vi "Create Response.vi"(8 "error in (no error)":errorcluster, 11 "message refnum in":T1 format="%.0x") -> (0 "error out":errorcluster, 2 "response refnum":T1=18446744073709551615 format="%.0x", 3 "message refnum out":T1 format="%.0x")   [LabVIEW 2020, in "Instrument Addon Scripting API.lvlib"]
doc: "Creates a Response section to the specified message. An error will occur if the refnum does not match an existing message."
uses:
  Instrument Addon Scripting API.lvlib
  <vilib>/NI VeriStand/Custom Device API/Custom Device Item Ref.ctl
  <vilib>/NI VeriStand/Custom Device API/Custom Device API.lvlib
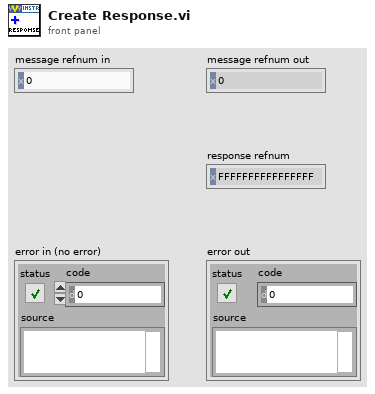
[diagram p1: front panel]
types:
  T1 = typedef "Custom Device API.lvlib/Custom Device Item Ref.ctl" = u64
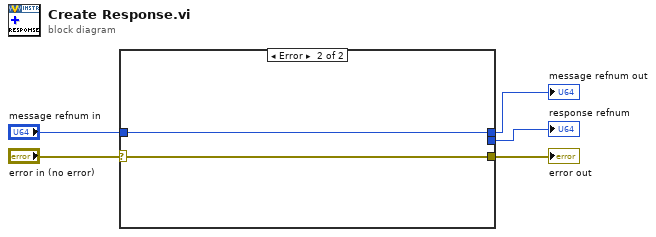
[diagram p0: block diagram]
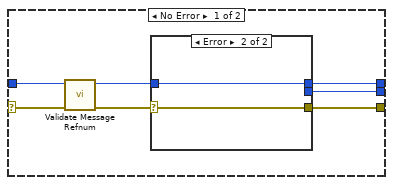
[diagram p2: hidden frame]
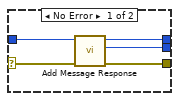
[diagram p3: hidden frame]
diagram:
  n1 = case shown="Error" "error in (no error)" {
    selector: "error in (no error)" -> [w12 w20]
    tunnel: "message refnum in" -> [w10 w21]
    tunnel: [w8 w21] -> w3
    tunnel: [w7 _] -> w2
    tunnel: [w6 w20] -> w1
    frame No Error {
      n2 = call "Validate Message Refnum.vi"("error in (no error)"=w12, "Message in"=w10) -> ("error out"=w11:errorcluster, "Message out"=w9:T1)  [unwired: 8 in]
      n3 = case shown="Error" w11 {
        selector: w11 -> [w17 w18]
        tunnel: w9 -> [w16 w19]
        tunnel: [w15 w19] -> w8
        tunnel: [w14 _] -> w7
        tunnel: [w13 w18] -> w6
        frame No Error {
          n4 = call "Add Message Response.vi"("Error In"=w17, "Message Refnum In"=w16) -> ("Error Out"=w13:errorcluster, "Response Section Ptr"=w14:T1, "Message Refnum Out"=w15:T1)  [unwired: 7 in]
        }
        frame Error {
        }
      }
    }
    frame Error {
    }
  }
  "message refnum out" <- w3
  "response refnum" <- w2
  "error out" <- w1
